vi "New Modify-Row and Delete.vi"() -> ()   [LabVIEW 2020]
uses:
  LabVIEW/g_ar_toolkit.common/Image Size (Integer).ctl
  LabVIEW/g_ar_toolkit.image/ARGB Colour.ctl
  LabVIEW/g_ar_toolkit.image/NewImageARGB.vi
  LabVIEW/g_ar_toolkit.image/NewImageARGB.vi/3321fa97-f432-4e1e-8db9-a0df79aed21b.vi
  LabVIEW/g_ar_toolkit.image/DrawImageToPictureARGB.vi/8cd07b1b-062e-4fe4-9e87-2eb3dc89fe0e.vi
  LabVIEW/g_ar_toolkit.common/Module Path.vi
  <vilib>/Utility/error.llb/Error Cluster From Error Code.vi
  LabVIEW/g_ar_toolkit.image/g_ar_toolkit.image.lvlib
  LabVIEW/g_ar_toolkit.common/g_ar_toolkit.common.lvlib
panel:
  in  "error in (no error)":errorcluster
  out "error out":errorcluster
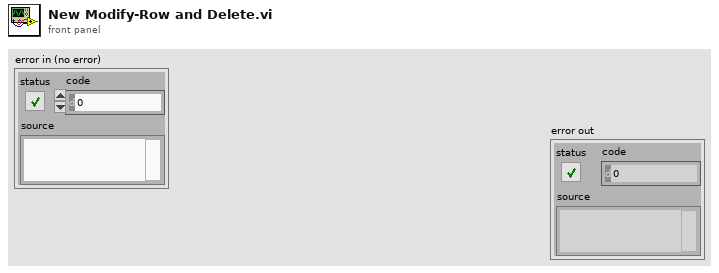
[diagram p1: front panel]
types:
  T1 = typedef "g_ar_toolkit.common.lvlib/Image Size (Integer).ctl" = cluster{"Width":u16, "Height":u16}
  T2 = typedef "g_ar_toolkit.image.lvlib/ARGB Image.ctl" = refnum<data-value>
  T3 = typedef "g_ar_toolkit.image.lvlib/ARGB Colour.ctl" = cluster{"Alpha":u8, "RGB":u32}
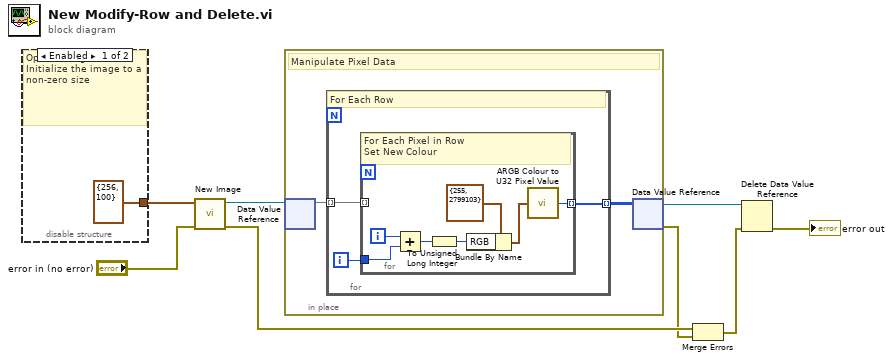
[diagram p0: block diagram]
diagram:
  n1 = disable-structure shown="Enabled" {
    disable-tunnel: [T1 {"Width"=256, "Height"=100} ("Preallocated Image Size (Default: 0,0)") _] -> w8
    frame Enabled {
      # "Optional Argument -\nInitialize the image to a non-zero size"
    }
    frame Disabled {
    }
  }
  n2 = call-poly "New Image.vi"("error in (no error)"="error in (no error)", "Preallocated Image Size (Default: 0,0)"=w8) -> ("error out"=w6:errorcluster, "New ARGB Image"=w7:T2)  [unwired: 8 in]
  n3 = in-place "In Place Element Structure" {
    # "Manipulate Pixel Data"
    n4 = in-place-dvr #1(w7) -> (w11:u32[][])  [unwired: 1 out]
    n5 = for {
      tunnel: w11 -> [w14] mode=indexing
      tunnel: [w13] -> w10 mode=indexing
      i -> [w12]
      # "For Each Row"
      n6 = for {
        tunnel: w14 -> [_] mode=indexing
        tunnel: [w20] -> w13 mode=indexing
        tunnel: w12 -> [w15]
        i -> [w18]
        # "For Each Pixel in Row\nSet New Colour"
        n7 = Add(x=w18, y=w15) -> (x+y=w16:i32)
        n8 = To Unsigned Long Integer(number=w16) -> (unsigned 32bit integer=w17:u32)
        n9 = Bundle By Name(cluster=T3 {"Alpha"=255, "RGB"=2799103} ("ARGB Colour"), "RGB"=w17) -> (w19:T3)
        n10 = call "ARGB Colour to U32 Pixel Value.vi"("ARGB Colour"=w19) -> ("U32 Colour"=w20:u32)
      }
    }
    n11 = in-place-dvr #1(w10) -> (w2:T2, w5:errorcluster)
  }
  n12 = Merge Errors(w6, w5) -> (w4:errorcluster)
  n13 = Delete Data Value Reference(data value reference=w2, error in=w4) -> (error out=→"error out":errorcluster)  [unwired: 1 out]
